vi "An_sync_block_sort_New.vi"(6 "BSA 2":dbl[][](array[numeric]) format="%.3f", 9 "BSA 1":dbl[][](array[numeric]) format="%.3f") -> (0 "Analogue Sync Index":i32[](array[numeric]), 1 "BSA 2 Sync":dbl[][](array[numeric]) format="%.3f", 3 "BSA 1 Sync":dbl[][](array[numeric]) format="%.3f", 4 "No of good samples":i32=1, 5 "No of slips":i32=1)   [LabVIEW 2010]
uses:
  Globals/LDA_meas_global_1.vi
  Globals/LDA_meas_global_2.vi
panel:
  out "Output":dbl[](graph)
  out "Input":dbl[](graph)
  out "Slipped":bool
  out "TIME MARGIN":dbl format="%.2f"
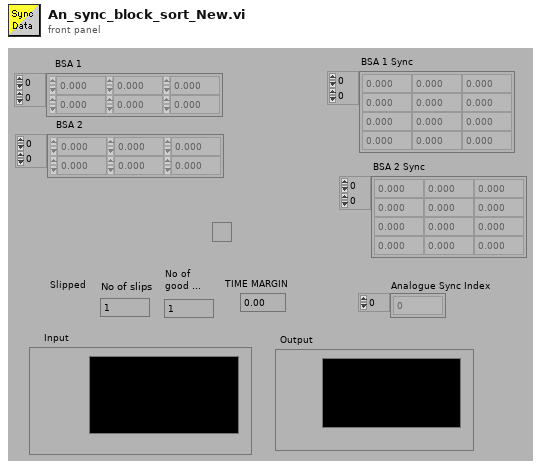
[diagram p1: front panel]
types:
  T1 = cluster{"Arrival time clock":enum16{"External", "Internal"}, "Clock source":enum16{"Slave", "Master", "Private"}, "Coincidence":enum16{"Slave", "Master", "Private"}}
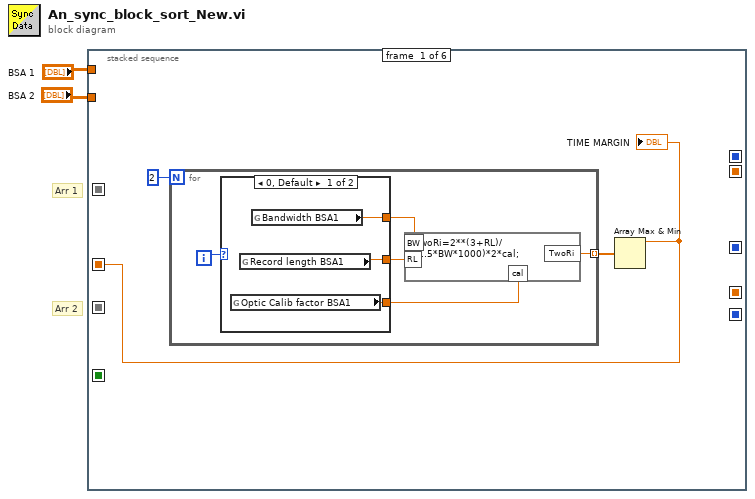
[diagram p0: block diagram]
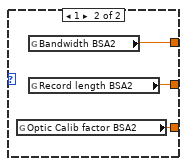
[diagram p2: hidden frame]
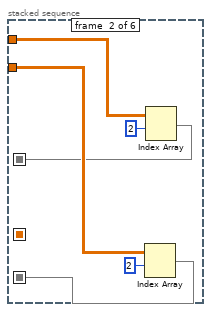
[diagram p3: hidden frame]
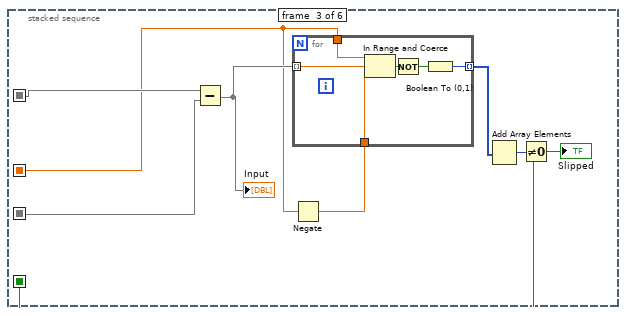
[diagram p4: hidden frame]
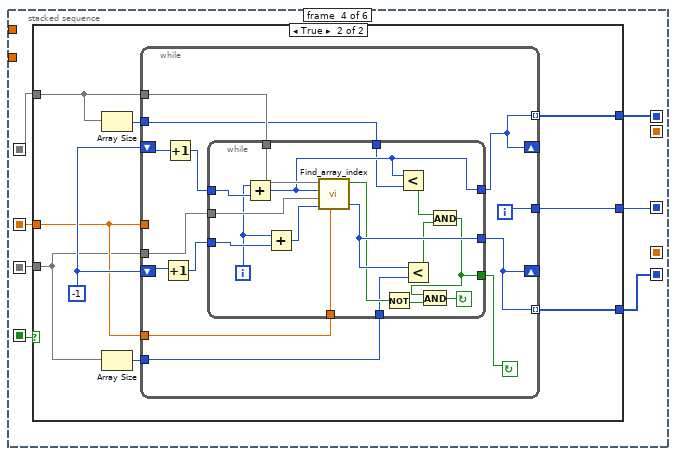
[diagram p5: hidden frame]
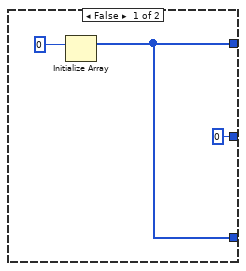
[diagram p6: hidden frame]
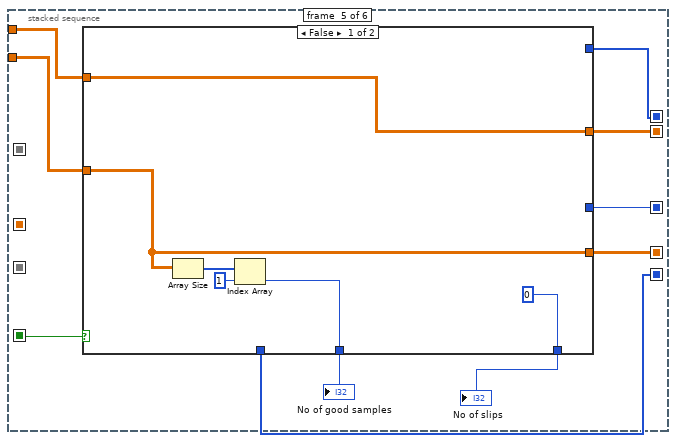
[diagram p7: hidden frame]
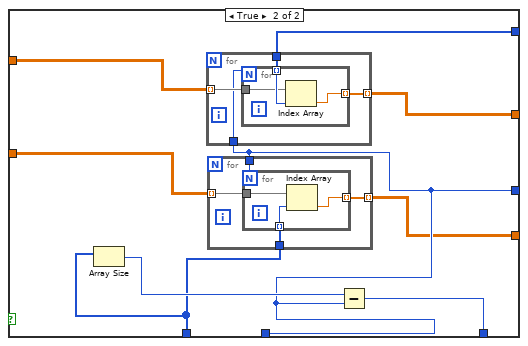
[diagram p8: hidden frame]
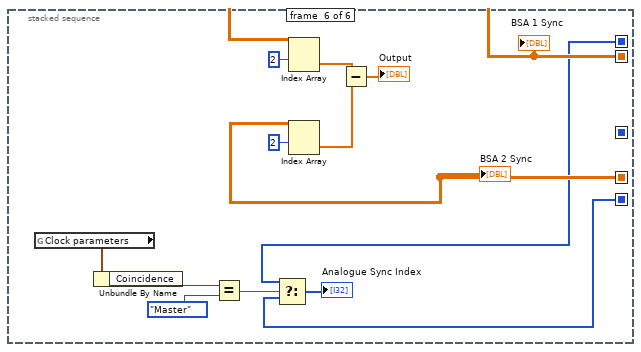
[diagram p9: hidden frame]
diagram:
  # "Arr 1"
  # "Arr 2"
  n1 = stacked-sequence {
    seq-local: [_ _ _ w43 _ _] -> [_ _ _ _ w94 w127]
    seq-local: [_ _ _ w42 _ _] -> [_ _ _ _ w95 w126]
    seq-local: [_ _ w28 _ _ _] -> [_ _ _ w41 w86 _]
    seq-local: [_ _ _ _ w88 _] -> [_ _ _ _ _ w135]
    seq-local: [_ w18 _ _ _ _] -> [_ _ w24 w40 _ _]
    seq-local: [_ w17 _ _ _ _] -> [_ _ w25 w39 _ _]
    seq-local: [_ _ _ w37 _ _] -> [_ _ _ _ w91 _]
    seq-local: [_ _ _ _ w87 _] -> [_ _ _ _ _ w132]
    seq-local: [w4 _ _ _ _ _] -> [_ _ w23 w38 _ _]
    tunnel: "BSA 1" -> [_ w22 _ _ w90 _]
    tunnel: "BSA 2" -> [_ w19 _ _ w89 _]
    frame #0 {
      n2 = for {
        N: 2 -> [_]
        tunnel: [w10] -> w5 mode=indexing
        i -> [w6]
        n3 = case shown="0, Default" w6 {
          tunnel: [w13 w16] -> w7
          tunnel: [w12 w15] -> w9
          tunnel: [w11 w14] -> w8
          frame 0, Default {
            n4 = global read "LDA_meas_global_1.vi" "Optic Calib factor BSA1"() -> (w13:dbl)
            n5 = global read "LDA_meas_global_1.vi" "Record length BSA1"() -> (w12:dbl)
            n6 = global read "LDA_meas_global_1.vi" "Bandwidth BSA1"() -> (w11:dbl)
          }
          frame 1 {
            n7 = global read "LDA_meas_global_2.vi" "Optic Calib factor BSA2"() -> (w16:dbl)
            n8 = global read "LDA_meas_global_2.vi" "Bandwidth BSA2"() -> (w14:dbl)
            n9 = global read "LDA_meas_global_2.vi" "Record length BSA2"() -> (w15:dbl)
          }
        }
        n10 = formula code="TwoRi=2**(3+RL)/(1.5*BW*1000)*2*cal;"("BW"=w8, "RL"=w9, "cal"=w7) -> ("TwoRi"=w10:dbl)
      }
      n11 = Array Max & Min(array=w5) -> (max value=w4:dbl)  [unwired: 3 out]
      "TIME MARGIN" <- w4
    }
    frame #1 {
      n12 = Index Array(array=w19, index (row)=2 ("Index")) -> (element=w17:dbl[])  [unwired: 1 in]
      n13 = Index Array(array=w22, index (row)=2 ("Index")) -> (element=w18:dbl[])  [unwired: 1 in]
    }
    frame #2 {
      n14 = Subtract(x=w24, y=w25) -> (x-y=w26:dbl[])
      "Input" <- w26
      n15 = Negate(x=w23) -> (-x=w30:dbl)
      n16 = for {
        tunnel: w23 -> [w36]
        tunnel: w30 -> [w35]
        tunnel: w26 -> [w34] mode=indexing
        tunnel: [w32] -> w27 mode=indexing
        n17 = In Range and Coerce(upper limit=w36, x=w34, lower limit=w35) -> (In Range?=w31:bool)  [unwired: 1 out]
        n18 = Not(x=w31) -> (.not. x?=w33:bool)
        n19 = Boolean To (0,1)(Boolean=w33) -> (0, 1=w32:i16)
      }
      n20 = Add Array Elements(numeric array=w27) -> (sum=w29:i16)
      n21 = Not Equal To 0?(x=w29) -> (x != 0?=w28:bool)
      "Slipped" <- w28
    }
    frame #3 {
      n22 = case shown="True" w41 {
        tunnel: w39 -> [_ w48]
        tunnel: w40 -> [_ w51]
        tunnel: [w45 w54] -> w43
        tunnel: [w45 w53] -> w42
        tunnel: w38 -> [_ w49]
        tunnel: [0 w52] -> w37
        frame False {
          n23 = Initialize Array(0) -> (w45:i32[])  [unwired: 1 out]
        }
        frame True {
          w55 = -1
          n24 = Array Size(array=w51) -> (size(s)=w50:i32)
          n25 = Array Size(array=w48) -> (size(s)=w47:i32)
          n26 = while {
            tunnel: w47 -> [w56]
            tunnel: w49 -> [w64]
            tunnel: w50 -> [w58]
            tunnel: [w66] -> w52
            tunnel: w49 -> [_]
            tunnel: [w62] -> w54 mode=indexing
            tunnel: [w59] -> w53 mode=indexing
            shift-left: w55 -> [w68]
            shift-right: [w59] -> _
            shift-left: w55 -> [w67]
            shift-right: [w62] -> _
            tunnel: w48 -> [w61]
            tunnel: w51 -> [w65]
            i -> [w66]
            stop <- w57 continue-if-true
            n27 = Increment(x=w68) -> (x+1=w60:i32)
            n28 = Increment(x=w67) -> (x+1=w63:i32)
            n29 = while {
              tunnel: w56 -> [w69]
              tunnel: [w71] -> w57
              tunnel: w58 -> [w70]
              tunnel: w65 -> [w79]
              tunnel: w64 -> [w80]
              tunnel: [w77] -> w59
              tunnel: [w78] -> w62
              tunnel: w61 -> [w83]
              tunnel: w60 -> [w84]
              tunnel: w63 -> [w85]
              i -> [w82]
              stop <- w72 continue-if-true
              n30 = Add(x=w82, y=w85) -> (x+y=w78:i32)
              n31 = Add(x=w82, y=w84) -> (x+y=w81:i32)
              n32 = call "Find_array_index.vi"("TIME MARGIN"=w80, "AT 2 index"=w81, "AT 2 array"=w83, "AT 1 index"=w78, "AT 1 array"=w79) -> ("AT 2 index out"=w77:i32, "Found matching Element in array 2"=w74:bool)  [unwired: 4 out]
              n33 = Not(x=w74) -> (.not. x?=w73:bool)
              n34 = Less?(x=w78, y=w70) -> (x < y?=w75:bool)
              n35 = Less?(x=w77, y=w69) -> (x < y?=w76:bool)
              n36 = And(x=w75, y=w76) -> (x .and. y?=w71:bool)
              n37 = And(x=w71, y=w73) -> (x .and. y?=w72:bool)
            }
          }
        }
      }
    }
    frame #4 {
      n38 = case shown="False" w86 {
        tunnel: w94 -> [_ w110]
        tunnel: w95 -> [_ w104]
        tunnel: [w96 w107] -> w93
        tunnel: [0 w108] -> w92
        tunnel: w91 -> [_ w107]
        tunnel: w90 -> [w100 w106]
        tunnel: w89 -> [w97 w105]
        tunnel: [w100 w103] -> w88
        tunnel: [w97 w102] -> w87
        frame False {
          n39 = Array Size(array=w97) -> (size(s)=w99:i32[])
          n40 = Index Array(array=w99, index=1 ("Index")) -> (element=w96:i32)
        }
        frame True {
          n41 = Array Size(array=w104) -> (size(s)=w109:i32)
          n42 = for {
            tunnel: w110 -> [w121]
            tunnel: w106 -> [w120] mode=indexing
            tunnel: [w119] -> w103 mode=indexing
            tunnel: w107 -> [w118]
            n43 = for {
              N: w118 -> [_]
              tunnel: w121 -> [w124] mode=indexing
              tunnel: w120 -> [w123]
              tunnel: [w122] -> w119 mode=indexing
              n44 = Index Array(array=w123, index=w124) -> (element=w122:dbl)
            }
          }
          n45 = for {
            tunnel: w105 -> [w114] mode=indexing
            tunnel: w104 -> [w113]
            tunnel: [w112] -> w102 mode=indexing
            tunnel: w107 -> [w111]
            n46 = for {
              N: w111 -> [_]
              tunnel: w114 -> [w117]
              tunnel: w113 -> [w116] mode=indexing
              tunnel: [w115] -> w112 mode=indexing
              n47 = Index Array(array=w117, index=w116) -> (element=w115:dbl)
            }
          }
          n48 = Subtract(x=w109, y=w107) -> (x-y=w108:i32)
        }
      }
      "No of slips" <- w92
      "No of good samples" <- w93
    }
    frame #5 {
      n49 = global read "LDA_meas_global_1.vi" "Clock parameters"() -> (w130:T1)
      n50 = Unbundle By Name(w130) -> ("Coincidence"=w129:enum16{"Slave", "Master", "Private"})
      n51 = Equal?(x=w129, y=enum16{"Slave", "Master", "Private"}."Master") -> (x = y?=w128:bool)
      n52 = Select(t=w127, s=w128, f=w126) -> (s? t:f=→"Analogue Sync Index":i32[])
      n53 = Index Array(array=w135, index (row)=2 ("Index")) -> (element=w138:dbl[])  [unwired: 1 in]
      n54 = Index Array(array=w132, index (row)=2 ("Index")) -> (element=w136:dbl[])  [unwired: 1 in]
      n55 = Subtract(x=w138, y=w136) -> (x-y=→"Output":dbl[])
      "BSA 1 Sync" <- w135
      "BSA 2 Sync" <- w132
    }
  }
